vi "Initialize.vi"(8 "error in (no error)":errorcluster, 11 "Microscope in":refnum<class "Microscope.lvclass">) -> (0 "error out":errorcluster, 3 "Microscope out":refnum<class "Microscope.lvclass">)   [LabVIEW 2020, in "Microscope.lvlib" / "Microscope.lvclass"]
uses:
  Microscope.lvclass
  Component/Device/Device/Device.lvclass
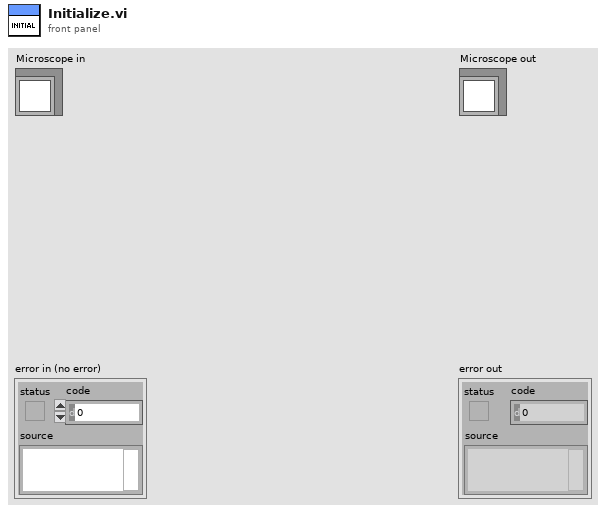
[diagram p1: front panel]
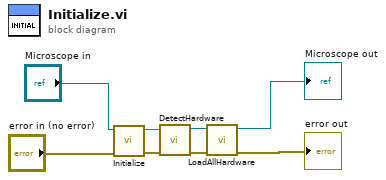
[diagram p0: block diagram]
diagram:
  n1 = call-parent "Initialize.vi"("error in (no error)"="error in (no error)", "Device in"="Microscope in") -> ("error out"=w8:errorcluster, "Device out"=w4:refnum<class "Microscope.lvclass">)  [unwired: 8 in]
  n2 = call-dynamic "DetectHardware.vi"("error in (no error)"=w8, "Microscope in"=w4) -> ("error out"=w5:errorcluster, "Microscope out"=w2:refnum<class "Microscope.lvclass">)  [unwired: 8 in]
  n3 = call-dynamic "LoadAllHardware.vi"("error in (no error)"=w5, "Microscope in"=w2) -> ("error out"=→"error out":errorcluster, "Microscope out"=→"Microscope out":refnum<class "Microscope.lvclass">)  [unwired: 8 in]
